vi "Test Stock Table - Animate - 02.vi"(8 "error in (no error)":errorcluster, 11 "TestCase in":refnum<class "TestCase.lvclass">) -> (0 "error out":errorcluster, 3 "TestCase out":refnum<class "TestCase.lvclass">)   [LabVIEW 2011, in "test.lvclass"]
uses:
  test.lvclass
  <vilib>/addons/_JKI Toolkits/VI Tester/TestCase.llb/TestCase.lvclass
  <vilib>/Utility/miscctls.llb/LVRowAndColumnTypeDef.ctl
panel:
  in  "Table":string[][](table)
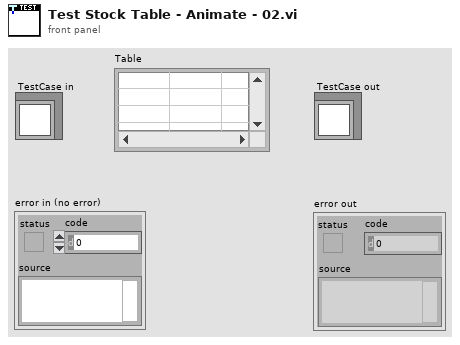
[diagram p1: front panel]
types:
  T1 = typedef "LVRowAndColumnTypeDef.ctl" = cluster{"Row":i32, "Column":i32}
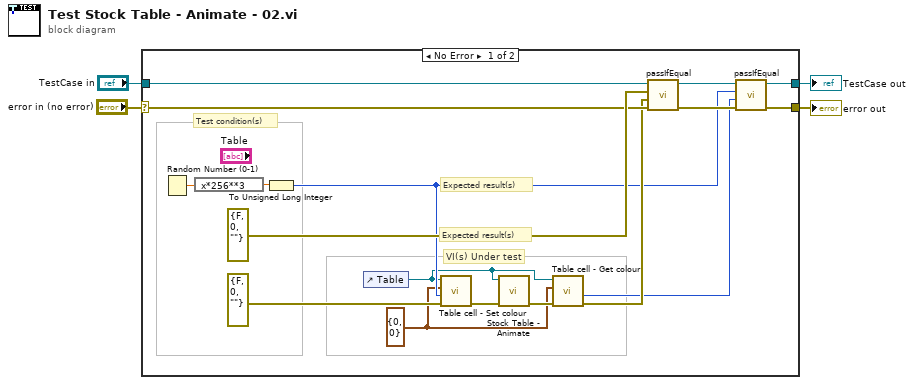
[diagram p0: block diagram]
diagram:
  n1 = case shown="No Error" "error in (no error)" {
    selector: "error in (no error)" -> [w19 w22]
    tunnel: "TestCase in" -> [w20 w23]
    tunnel: [w17 w23] -> w3
    tunnel: [w18 w22] -> w2
    frame No Error {
      w5 = T1 {"Row"=0, "Column"=0} ("Table Active Cell")
      # "Expected result(s)"
      # "Expected result(s)"
      # "Test condition(s)"
      # "VI(s) Under test"
      n2 = Random Number (0-1)() -> (number: 0 to 1=w14:dbl)
      n3 = expression code="x*256**3"(w14) -> (w13:dbl)
      n4 = To Unsigned Long Integer(number=w13) -> (unsigned 32bit integer=w7:u32)
      n5 = control-ref of="Table"() -> (w6:refnum<vi>)
      n6 = call "Table cell - Set colour.vi"("error in"=errorcluster {"status"=FALSE, "code"=0, "source"=""} ("error in (no error)"), "Active Cell Background Color"=w7, "Table Active Cell"=w5, "Table Reference"=w6) -> ("error out"=w9:errorcluster)  [unwired: 7 in]
      n7 = call "Stock Table - Animate.vi"("error in"=w9, "Table Reference"=w6) -> ("error out"=w12:errorcluster)  [unwired: 9 in]
      n8 = call "Table cell - Get colour.vi"("error in"=w12, "Table Active Cell"=w5, "Table Reference"=w6) -> ("error out"=w11:errorcluster, "Active Cell Background Color"=w8:u32)  [unwired: 7 in]
      n9 = call-dynamic "passIfEqual.vi"("error in (no error)"=w19, "y"=w11, "x"=errorcluster {"status"=FALSE, "code"=0, "source"=""} ("error in (no error)"), "TestCase in"=w20) -> ("error out"=w15:errorcluster, "TestCase out"=w16:refnum<class "TestCase.lvclass">)  [unwired: 6 in]
      n10 = call-dynamic "passIfEqual.vi"("error in (no error)"=w15, "y"=w8, "x"=w7, "TestCase in"=w16) -> ("error out"=w18:errorcluster, "TestCase out"=w17:refnum<class "TestCase.lvclass">)  [unwired: 6 in]
    }
    frame Error {
    }
  }
  "TestCase out" <- w3
  "error out" <- w2
